vi "rename_document.vi"(10 "did":string, 11 "Name":string) -> (1 "path":string, 2 "payload":string, 3 "Method":string)   [LabVIEW 2019]
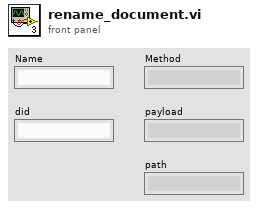
[diagram p1: front panel]
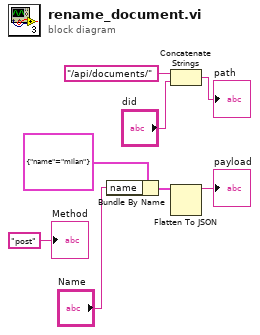
[diagram p0: block diagram]
diagram:
  n1 = Bundle By Name(cluster=cluster{"name":string} {"name"="milan"}, "name"="Name") -> (w2:cluster{"name":string})
  n2 = Concatenate Strings("/api/documents/" ("payload"), "did") -> (→"path":string)
  n3 = Flatten To JSON(anything=w2) -> (JSON string=→"payload":string)  [unwired: 2 in, 1 out]
  "Method" <- "post" ("Method")
